vi "Send UserInfo.vi"(5 "Message Type":refnum<class "UserInfo Msg.lvclass">, 7 "Message Priority (Normal)":T3=enum."Normal", 8 "error in (no error)":errorcluster, 10 "LoginResponse":cluster{"UserInfo":T1, "PassWordExists？":bool}, 11 "Message Enqueuer":refnum<class "Message Enqueuer.lvclass">) -> (0 "error out":errorcluster, 3 "Message Enqueuer out":refnum<class "Message Enqueuer.lvclass">)   [LabVIEW 2019, in "UserManagement.lvlib" / "UserInfo Msg.lvclass"]
doc: "This VI sends the message to an actor."
uses:
  UserInfo Msg.lvclass
  <vilib>/ActorFramework/Message Enqueuer/Message Enqueuer.lvclass
  <vilib>/ActorFramework/Message Enqueuer/Message Priority.ctl
  C:/Program Files (x86)/National Instruments/LabVIEW 2019/vi.lib/ActorFramework/Message/Message.lvclass
  UserManagement/UserInfo.ctl
  UserManagement/Permission.ctl
  UserInfo Msg.lvclass/UserInfo Msg.ctl
  <vilib>/ActorFramework/Message Enqueuer/Message Enqueuer.lvclass/Message Enqueuer.ctl
  <vilib>/ActorFramework/Message Priority Queue/Priority Enqueue.vi
  UserManagement/UserManagement.lvclass
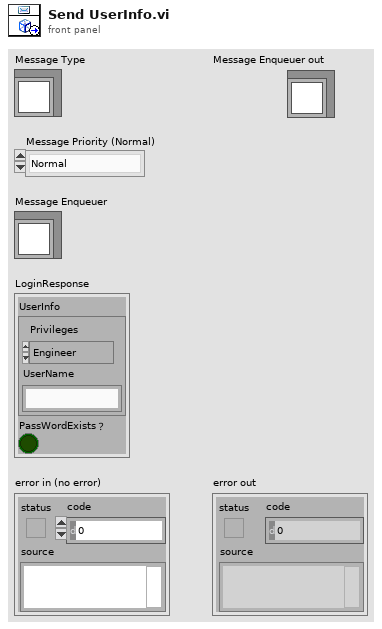
[diagram p1: front panel]
types:
  T1 = typedef "UserManagement.lvlib/UserManagement.lvclass/UserInfo.ctl" = cluster{"Privileges":T2, "UserName":string}
  T2 = typedef "UserManagement.lvlib/UserManagement.lvclass/Permission.ctl" = enum16{"Engineer", "Technical", "Operator"}
  T3 = typedef "Actor Framework.lvlib/Message Enqueuer.lvclass/Message Priority.ctl" = enum16{"Low", "Normal", "High"}
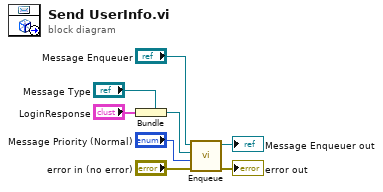
[diagram p0: block diagram]
diagram:
  n1 = Bundle(cluster="Message Type", "LoginResponse") -> (w4:refnum<class "UserInfo Msg.lvclass">)
  n2 = call <vilib>:"Enqueue.vi"("error in (no error)"="error in (no error)", "Message Priority (Normal)"="Message Priority (Normal)", "Message"=w4, "Message Enqueuer in"="Message Enqueuer") -> ("error out"=→"error out":errorcluster, "Message Enqueuer out"=→"Message Enqueuer out":refnum<class "Message Enqueuer.lvclass">)  [unwired: 6 in]
